vi "subReplaceSourceLibaryWithBuiltLib.vi"(8 "error in (no error)":errorcluster, 10 "ProjectItem in":refnum<class "ProjectItem.lvclass">, 11 "BuildManager in":refnum<class "BuildManager.lvclass">) -> (0 "error out":errorcluster, 3 "BuildManager out":refnum<class "BuildManager.lvclass">)   [LabVIEW 2019, in "SolutionBuilder.lvlib" / "BuildManager.lvclass"]
uses:
  BuildManager.lvclass
  ProjectItem/ProjectItem.lvclass
  ProjectItem/ProjectItem.lvclass/ProjectItem.ctl
  BuildManager.lvclass/BuildManager.ctl
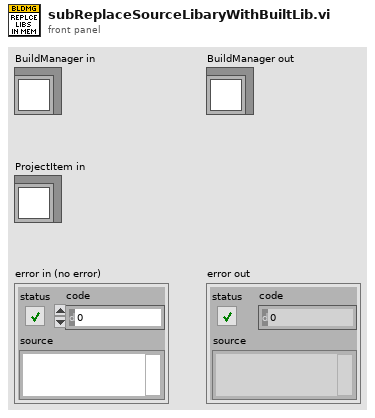
[diagram p1: front panel]
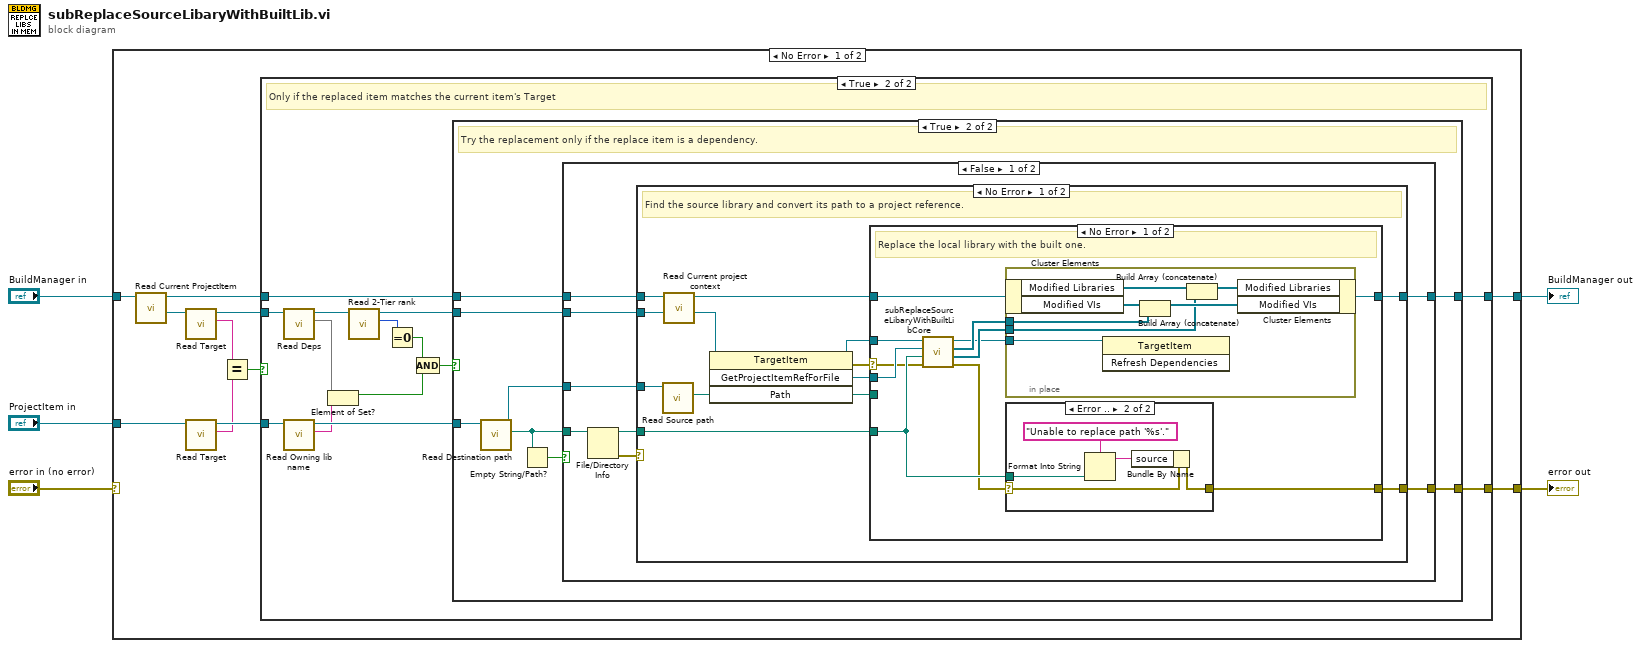
[diagram p0: block diagram]
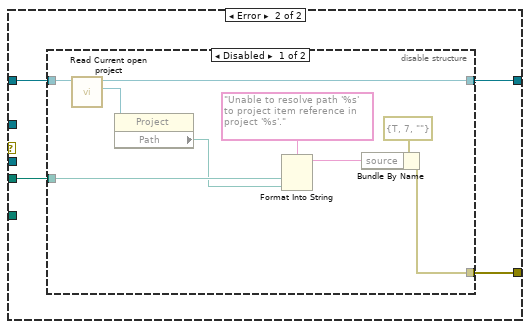
[diagram p5: hidden frame]
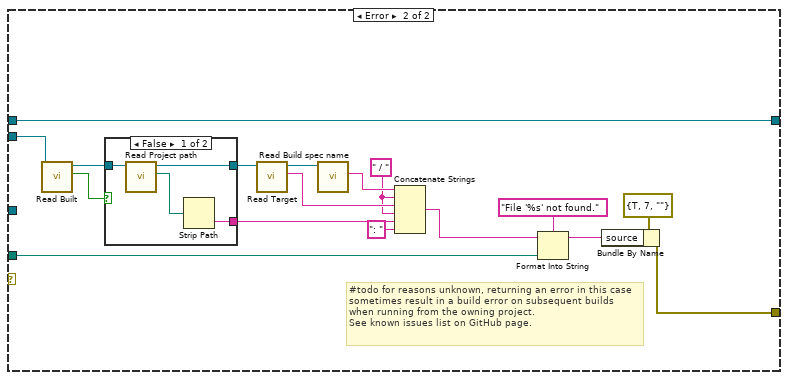
[diagram p7: hidden frame]
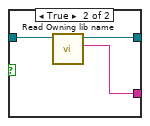
[diagram p8: hidden frame]
diagram:
  n1 = case shown="No Error" "error in (no error)" {
    selector: "error in (no error)" -> [_ w125]
    tunnel: [w16 w124] -> w5
    tunnel: "BuildManager in" -> [w13 w124]
    tunnel: "ProjectItem in" -> [w9 _]
    tunnel: [w15 w125] -> w1
    frame No Error {
      n2 = call-dynamic "Read Current ProjectItem.vi"("BuildManager in"=w13) -> ("Current ProjectItem"=w12:refnum<class "ProjectItem.lvclass">, "BuildManager out"=w14:refnum<class "BuildManager.lvclass">)  [unwired: 7 in, 2 out]
      n3 = call "Read Target.vi"("ProjectItem in"=w12) -> ("Target"=w8:string, "ProjectItem out"=w11:refnum<class "ProjectItem.lvclass">)  [unwired: 9 in]
      n4 = call "Read Target.vi"("ProjectItem in"=w9) -> ("Target"=w7:string, "ProjectItem out"=w10:refnum<class "ProjectItem.lvclass">)  [unwired: 9 in]
      n5 = Equal?(x=w8, y=w7) -> (x = y?=w6:bool)
      n6 = case shown="True" w6 {
        tunnel: [w17 w31] -> w16
        tunnel: [_ w30] -> w15
        tunnel: w14 -> [w17 w29]
        tunnel: w11 -> [_ w19]
        tunnel: w10 -> [_ w18]
        frame False {
        }
        frame True {
          # "Only if the replaced item matches the current item's Target"
          n7 = call-dynamic "Read Deps.vi"("ProjectItem in"=w19) -> ("Deps"=w27:set{string}, "ProjectItem out"=w25:refnum<class "ProjectItem.lvclass">)  [unwired: 9 in]
          n8 = call-dynamic "Read Owning lib name.vi"("ProjectItem in"=w18) -> ("Owning lib name"=w26:string, "ProjectItem out"=w28:refnum<class "ProjectItem.lvclass">)  [unwired: 9 in]
          n9 = Element of Set?(10:w26, 11:w27) -> (3:w22:bool)
          n10 = call-dynamic "Read 2-Tier rank.vi"("ProjectItem in"=w25) -> ("2-Tier rank"=w24:u8, "ProjectItem out"=w20:refnum<class "ProjectItem.lvclass">)  [unwired: 9 in]
          n11 = Equal To 0?(x=w24) -> (x = 0?=w23:bool)
          n12 = Compound Arithmetic op=AND(w23, w22) -> (w21:bool)
          n13 = case shown="True" w21 {
            tunnel: [w32 w40] -> w31
            tunnel: [_ w36] -> w30
            tunnel: w29 -> [w32 w35]
            tunnel: w28 -> [_ w34]
            tunnel: w20 -> [_ w33]
            frame False {
            }
            frame True {
              # "Try the replacement only if the replace item is a dependency."
              n14 = call-dynamic "Read Destination path.vi"("ProjectItem in"=w34) -> ("Destination path"=w38:path, "ProjectItem out"=w37:refnum<class "ProjectItem.lvclass">)  [unwired: 9 in]
              n15 = Empty String/Path?(string/path=w38) -> (empty?=w39:bool)
              n16 = case shown="False" w39 {
                tunnel: w37 -> [w48 _]
                tunnel: w38 -> [w44 _]
                tunnel: w35 -> [w46 w123]
                tunnel: [w47 w123] -> w40
                tunnel: [w42 _] -> w36
                tunnel: w33 -> [w41 _]
                frame False {
                  n17 = File/Directory Info(path=w44) -> (path out=w45:path, error out=w43:errorcluster)  [unwired: 1 in, 5 out]
                  n18 = case shown="No Error" w43 {
                    tunnel: w48 -> [w59 _]
                    tunnel: [w57 w115] -> w47
                    tunnel: w46 -> [w55 w115]
                    tunnel: w45 -> [w52 w111]
                    tunnel: [w50 w110] -> w42
                    tunnel: w41 -> [w49 w105]
                    frame No Error {
                      # "Find the source library and convert its path to a project reference."
                      n19 = call-dynamic "Read Source path.vi"("ProjectItem in"=w59) -> ("Source path"=w51:path)  [unwired: 9 in, 1 out]
                      n20 = call-dynamic "Read Current project context.vi"("Current ProjectItem"=w49, "BuildManager in"=w55) -> ("Project context"=w53:refnum<vi>, "BuildManager out"=w54:refnum<class "BuildManager.lvclass">)  [unwired: 8 in]
                      n21 = invoke class="TargetItem" method="GetProjectItemRefForFile"(reference=w53, "Path"=w51) -> (reference out=w56:refnum<vi>, error out=w58:errorcluster, "GetProjectItemRefForFile"=w60:refnum<vi>)  [unwired: 2 in, 1 out]
                      n22 = case shown="No Error" w58 {
                        selector: w58 -> [w61 _]
                        tunnel: w60 -> [w71 _]
                        tunnel: w52 -> [w65 _]
                        tunnel: w54 -> [w70 w85]
                        tunnel: [w67 w86] -> w57
                        tunnel: w56 -> [w62 _]
                        tunnel: w51 -> [_ w88]
                        tunnel: [w66 w87] -> w50
                        frame No Error {
                          # "Replace the local library with the built one."
                          n23 = call "subReplaceSourceLibaryWithBuiltLibCore.vi"("error in (no error)"=w61, "path in"=w65, "GetProjectItemRefForFile"=w71, "TargetItem in"=w62) -> ("error out"=w64:errorcluster, "Modified Libraries"=w68:refnum<vi>[], "Modified VIs"=w69:refnum<vi>[], "TargetItem out"=w63:refnum<vi>)  [unwired: 4 in]
                          n24 = in-place {
                            in-place-border: w69 -> [w83]
                            in-place-border: w68 -> [w80]
                            in-place-border: w63 -> [w78]
                            n25 = in-place-cluster #1(w70) -> ("Modified Libraries"=w81:refnum<vi>[], "Modified VIs"=w84:refnum<vi>[])
                            n26 = invoke class="TargetItem" method="Refresh Dependencies"(reference=w78) -> ()  [unwired: 2 in, 3 out]
                            n27 = Build Array (concatenate)(w84, w83) -> (w82:refnum<vi>[])
                            n28 = Build Array (concatenate)(w81, w80) -> (w79:refnum<vi>[])
                            n29 = in-place-cluster #1("Modified Libraries"=w79, "Modified VIs"=w82) -> (w67:refnum<class "BuildManager.lvclass">)
                          }
                          n30 = case shown="Error .." w64 {
                            selector: w64 -> [w72 w73]
                            tunnel: [w72 w77] -> w66
                            tunnel: w65 -> [_ w75]
                            frame No Error {
                            }
                            frame Error {
                              n31 = Format Into String(format string="Unable to replace path '%s'.", w75) -> (resulting string=w74:string)  [unwired: 2 in, 1 out]
                              n32 = Bundle By Name(cluster=w73, "source"=w74) -> (w77:errorcluster)
                            }
                          }
                        }
                        frame Error {
                          n33 = disable-structure shown="Disabled" {
                            disable-tunnel: w88 -> [w94 _]
                            disable-tunnel: [w93 _] -> w87
                            disable-tunnel: [w92 w98] -> w86
                            disable-tunnel: w85 -> [w91 w98]
                            frame Disabled {
                              n34 = call-dynamic "Read Current open project.vi"("BuildManager in"=w91) -> ("Current open project"=w90:refnum<vi>, "BuildManager out"=w92:refnum<class "BuildManager.lvclass">)  [unwired: 9 in]
                              n35 = property class="Project"(reference=w90) -> ("Path"=w89:path)  [unwired: 1 in, 2 out]
                              n36 = Format Into String(format string="Unable to resolve path '%s' to project item reference in project '%s'.", w94, w89) -> (resulting string=w95:string)  [unwired: 2 in, 1 out]
                              n37 = Bundle By Name(cluster=errorcluster {"status"=TRUE, "code"=7, "source"=""} ("error out"), "source"=w95) -> (w93:errorcluster)
                            }
                            frame Enabled {
                            }
                          }
                        }
                      }
                    }
                    frame Error {
                      w102 = " / " ("string")
                      # "#todo for reasons unknown, returning an error in this case sometimes result in a build error on subsequent builds when running from the owning project.\nSee known issues list on GitHub page."
                      n38 = call-dynamic "Read Built.vi"("ProjectItem in"=w105) -> ("Built"=w107:bool, "ProjectItem out"=w108:refnum<class "ProjectItem.lvclass">)  [unwired: 9 in]
                      n39 = case shown="False" w107 {
                        tunnel: w108 -> [w119 w122]
                        tunnel: [w117 w120] -> w101
                        tunnel: [w116 w121] -> w106
                        frame False {
                          n40 = call-dynamic "Read Project path.vi"("ProjectItem in"=w119) -> ("Project path"=w118:path, "ProjectItem out"=w116:refnum<class "ProjectItem.lvclass">)  [unwired: 9 in]
                          n41 = Strip Path(path=w118) -> (name=w117:string)  [unwired: 1 out]
                        }
                        frame True {
                          n42 = call-dynamic "Read Owning lib name.vi"("ProjectItem in"=w122) -> ("Owning lib name"=w120:string, "ProjectItem out"=w121:refnum<class "ProjectItem.lvclass">)  [unwired: 9 in]
                        }
                      }
                      n43 = call "Read Target.vi"("ProjectItem in"=w106) -> ("Target"=w103:string, "ProjectItem out"=w109:refnum<class "ProjectItem.lvclass">)  [unwired: 9 in]
                      n44 = call-dynamic "Read Build spec name.vi"("ProjectItem in"=w109) -> ("Build spec name"=w104:string)  [unwired: 9 in, 1 out]
                      n45 = Concatenate Strings(w104, w102, w103, w102, w101, ": " ("string")) -> (w99:string)
                      n46 = Format Into String(format string="File '%s' not found.", initial string=w99, w111) -> (resulting string=w112:string)  [unwired: 1 in, 1 out]
                      n47 = Bundle By Name(cluster=errorcluster {"status"=TRUE, "code"=7, "source"=""} ("error out"), "source"=w112) -> (w110:errorcluster)
                    }
                  }
                }
                frame True {
                }
              }
            }
          }
        }
      }
    }
    frame Error {
    }
  }
  "BuildManager out" <- w5
  "error out" <- w1
